vi "Set Map Cache Directory.vi"(8 "Error In":errorcluster, 11 "Map Ref":refnum<k24>(container)) -> (0 "Error Out":errorcluster, 3 "Map Ref 2":refnum<k24>(container))   [LabVIEW 2014]
uses:
  C:/Robotic Systems/Products/AgFalcon/Software/Ground Station/Data/Mapping DLL/GMap.NET.WindowsForms.dll
  Data/Mapping DLL/GMap.NET.WindowsForms.dll
  C:/Robotic Systems/Products/AgFalcon/Software/Ground Station/Data/Mapping DLL/GMap.NET.Core.dll
  Data/Mapping DLL/GMap.NET.Core.dll
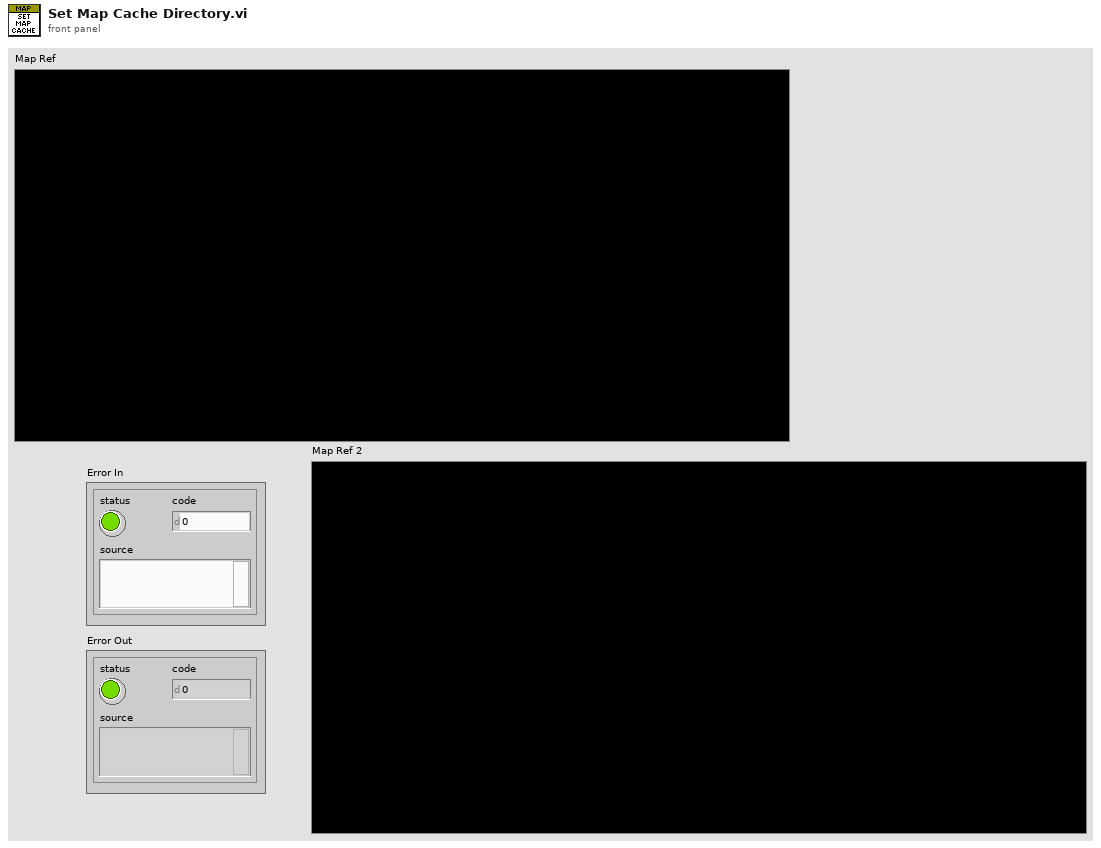
[diagram p1: front panel]
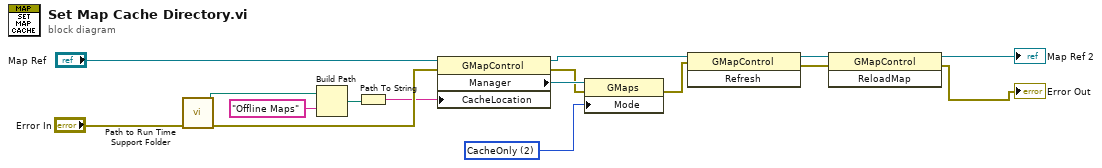
[diagram p0: block diagram]
diagram:
  w11 = 2 items=["ServerOnly", "ServerAndCache", "CacheOnly"] ("Mode")
  n1 = call "Path to Run Time Support Folder.vi"("Error In"="Error In") -> ("Error Out"=w8:errorcluster, "Path To Run Time Support Folder"=w15:path)  [unwired: 9 in]
  n2 = Build Path(base path=w15, name or relative path="Offline Maps") -> (appended path=w16:path)
  n3 = Path To String(path=w16) -> (string=w7:string)
  n4 = property class="GMapControl"(reference="Map Ref", error in=w8, "CacheLocation"=w7) -> (reference out=w6:refnum<k24>, error out=w9:errorcluster, "Manager"=w10:refnum<k24>)
  n5 = property class="GMaps"(reference=w10, error in=w9, "Mode"=w11) -> (error out=w5:errorcluster)  [unwired: 1 out]
  n6 = invoke class="GMapControl" method="Refresh"(reference=w6, error in=w5) -> (reference out=w4:refnum<k24>, error out=w3:errorcluster)  [unwired: 1 in, 1 out]
  n7 = invoke class="GMapControl" method="ReloadMap"(reference=w4, error in=w3) -> (reference out=→"Map Ref 2":refnum<k24>, error out=→"Error Out":errorcluster)  [unwired: 1 in, 1 out]
